vi "Example Enumerate.vi"() -> ()   [LabVIEW 2010]
uses:
  C:/tf/play/labview/Tinkerforge.dll
panel:
  out "events":string[](array[string])
  in  "stop":bool
  in  "port":i32=4223
  in  "host":string="localhost"
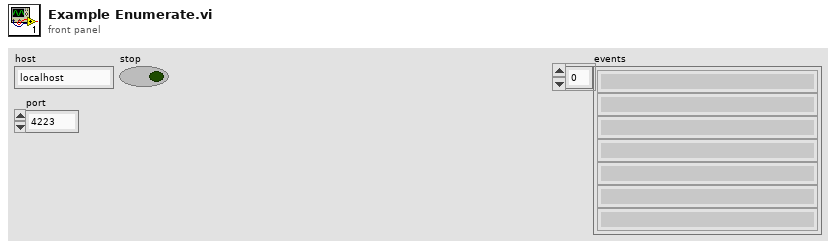
[diagram p1: front panel]
types:
  T1 = cluster{"uid":string, "connectedUid":string, "position":u16, "hardwareVersion":i16[], "firmwareVersion":i16[], "deviceIdentifier":i32, "enumerationType":i16}
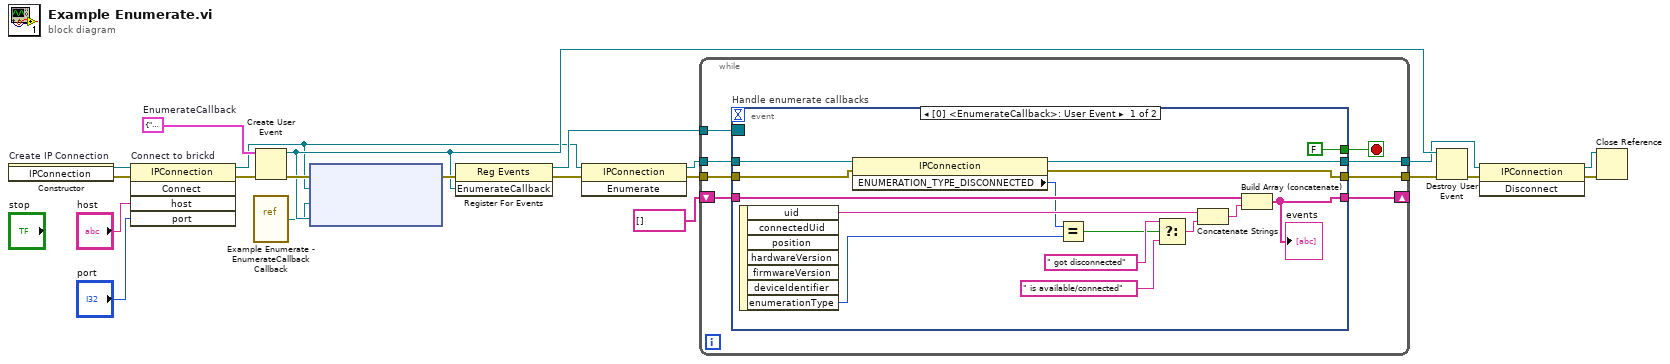
[diagram p0: block diagram]
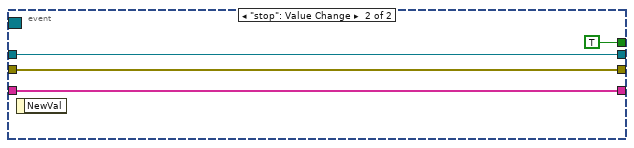
[diagram p2: hidden frame]
diagram:
  w10 = T1 {"uid"="", "connectedUid"="", "position"=0, "hardwareVersion"=[], "firmwareVersion"=[], "deviceIdentifier"=0, "enumerationType"=0}  # EnumerateCallback
  n1 = constructor on="Create IP Connection" class="IPConnection"() -> (reference out=w21:refnum<k24>, error out=w1:errorcluster)  [unwired: 3 in, 1 out]
  n2 = invoke on="Connect to brickd" class="IPConnection" method="Connect"(reference=w21, error in=w1, "host"="host", "port"="port") -> (reference out=w6:refnum<k24>, error out=w9:errorcluster)  [unwired: 1 in, 3 out]
  n3 = vi-ref "Example Enumerate - EnumerateCallback Callback.vi"() -> ("vi reference"=w7:refnum<vi>)
  n4 = Create User Event(user event datatype=w10, error in=w9) -> (user event=w12:refnum<user-event>, error out=w16:errorcluster)
  n5 = node ("Register Event Callback")(w16, w6, w7, w12) -> (w15:errorcluster)  [unwired: 1 in, 1 out]
  n6 = register-events(error in=w15, w12) -> (reference out=w14:refnum<event-registration>, error out=w11:errorcluster)  [unwired: 1 in]
  n7 = invoke class="IPConnection" method="Enumerate"(reference=w6, error in=w11) -> (reference out=w4:refnum<k24>, error out=w8:errorcluster)  [unwired: 1 in, 1 out]
  n8 = while {
    tunnel: w14 -> [w29]
    tunnel: [w28] -> w13
    tunnel: w8 -> [w27]
    shift-right: [w24] -> _
    shift-left: string[] [] -> [w25]
    tunnel: w4 -> [w23]
    tunnel: [w22] -> w3
    stop <- w26 stop-if-true
    n9 = event "Handle enumerate callbacks" shown="[0] <EnumerateCallback>: User Event" {
      selector: w29 -> [_ _]
      dyn-events: _ -> [_ _]
      timeout: _ -> [_ _]
      tunnel: [w35 w46] -> w28
      tunnel: w27 -> [w36 w46]
      tunnel: [FALSE TRUE] -> w26
      tunnel: w25 -> [w40 w47]
      tunnel: [w39 w47] -> w24
      tunnel: w23 -> [w37 w45]
      tunnel: [w33 w45] -> w22
      event User Event {
        n10 = event-data() -> ("uid"=w43:string, "enumerationType"=w31:i16)  [unwired: 1 in, 5 out]
        n11 = property class="IPConnection"(reference=w37, error in=w36) -> (reference out=w33:refnum<k24>, error out=w35:errorcluster, "ENUMERATION_TYPE_DISCONNECTED"=w30:i16)
        n12 = Equal?(x=w30, y=w31) -> (x = y?=w32:bool)
        n13 = Select(t=" got disconnected", s=w32, f=" is available/connected") -> (s? t:f=w38:string)
        n14 = Concatenate Strings(w43, w38) -> (w34:string)
        n15 = Build Array (concatenate)(w40, w34) -> (w39:string[])
        "events" <- w39
      }
      event "stop": Value Change {
        n16 = event-data() -> ()  [unwired: 1 in, 1 out]
      }
    }
  }
  n17 = Destroy User Event(user event=w12, error in=w13) -> (error out=w5:errorcluster)
  n18 = invoke class="IPConnection" method="Disconnect"(reference=w3, error in=w5) -> (reference out=w17:refnum<k24>, error out=w18:errorcluster)  [unwired: 1 in, 1 out]
  n19 = Close Reference(reference=w17, error in (no error)=w18) -> ()  [unwired: 1 out]
